vi "Configure Power Analysis (On Off).vi"(7 "Analysis Type (0: Turn On)":i32(ring) items=["Turn On", "Turn Off"], 8 "error in (no error)":errorcluster, 10 "Operation (0: Apply)":i32(ring) items=["Apply", "Exit", "Go to Next Step", "Test"], 11 "VISA resource name":refnum<visa-resource-name>) -> (0 "error out":errorcluster, 3 "VISA resource name out":refnum<visa-resource-name>)   [LabVIEW 2023, in "Keysight-DSQx3014T.lvlib"]
doc: "Configures turn on/off analysis test."
uses:
  Keysight-DSQx3014T.lvlib
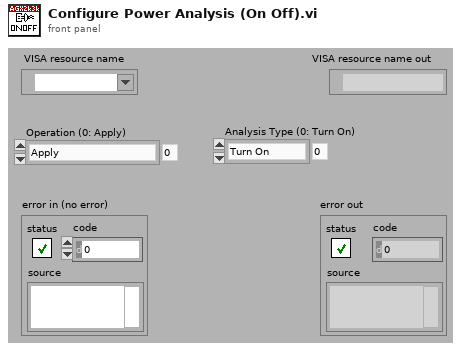
[diagram p1: front panel]
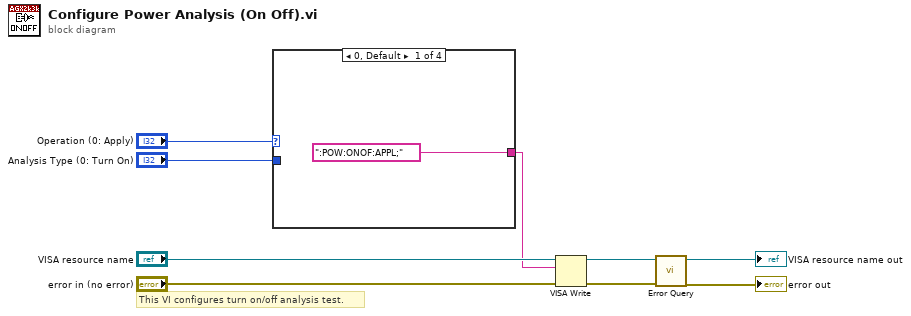
[diagram p0: block diagram]
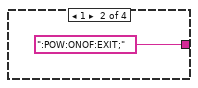
[diagram p2: hidden frame]
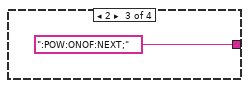
[diagram p3: hidden frame]
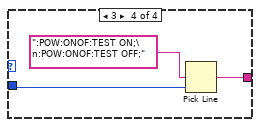
[diagram p4: hidden frame]
diagram:
  # "This VI configures turn on/off analysis test."
  n1 = case shown="0, Default" "Operation (0: Apply)" {
    tunnel: "Analysis Type (0: Turn On)" -> [_ _ _ w14]
    tunnel: [":POW:ONOF:APPL;" ":POW:ONOF:EXIT;" ":POW:ONOF:NEXT;" w13] -> w1
    frame 0, Default {
    }
    frame 1 {
    }
    frame 2 {
    }
    frame 3 {
      n2 = Pick Line(multi-line string=":POW:ONOF:TEST ON;\n:POW:ONOF:TEST OFF;", line index=w14) -> (output string=w13:string)  [unwired: 1 out]
    }
  }
  n3 = VISA Write(VISA resource name="VISA resource name", write buffer=w1, error in (no error)="error in (no error)") -> (VISA resource name out=w7:refnum<visa-resource-name>, error out=w6:errorcluster)  [unwired: 1 out]
  n4 = call "Error Query.vi"("error in (no error)"=w6, "VISA resource name"=w7) -> ("error out"=→"error out":errorcluster, "VISA resource name out"=→"VISA resource name out":refnum<visa-resource-name>)  [unwired: 8 out]
